vi "code to create file.vi"(0 "queue":refnum<queue>, 2 "Procesar datos en Matlab":bool, 9 "Path":path, 11 "error in (no error)":errorcluster) -> (4 "queue  out":refnum<queue>, 15 "error out":errorcluster)   [LabVIEW 2013]
doc: "This SubVI contain code to create file"
uses:
  bus to create file.ctl
  data simulation bus.ctl
  VoltElectrodo.ctl
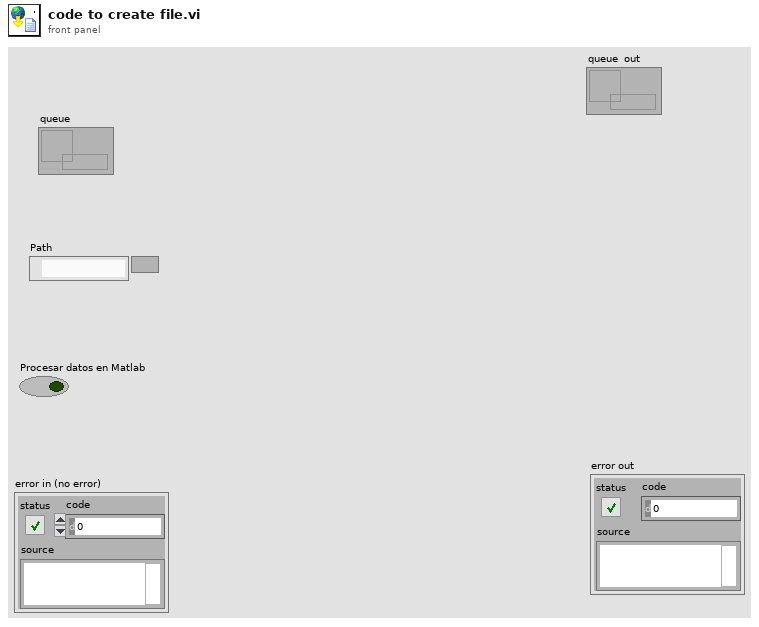
[diagram p1: front panel]
types:
  T1 = typedef "bus to create file.ctl" = cluster{"data simulation":T2, "Time":dbl, "volt":T3}
  T2 = typedef "data simulation bus.ctl" = cluster{"Flujo pulpa ":dbl, "Flujo agua lavado":dbl, "Flujo aire":dbl, "Flujo relave":dbl, "Altura capa de espuma":dbl, "Gas holdup":dbl, "% apertura valvula aire":dbl, "ref pulp":dbl}
  T3 = typedef "VoltElectrodo.ctl" = cluster{"V1":dbl, "V2":dbl, "V3":dbl, "V4":dbl, "V5":dbl, "V6":dbl, "V7":dbl, "V8":dbl}
  T4 = enum16{"open", "replace", "create", "open or create", "replace or create", "replace or create with confirmation"}
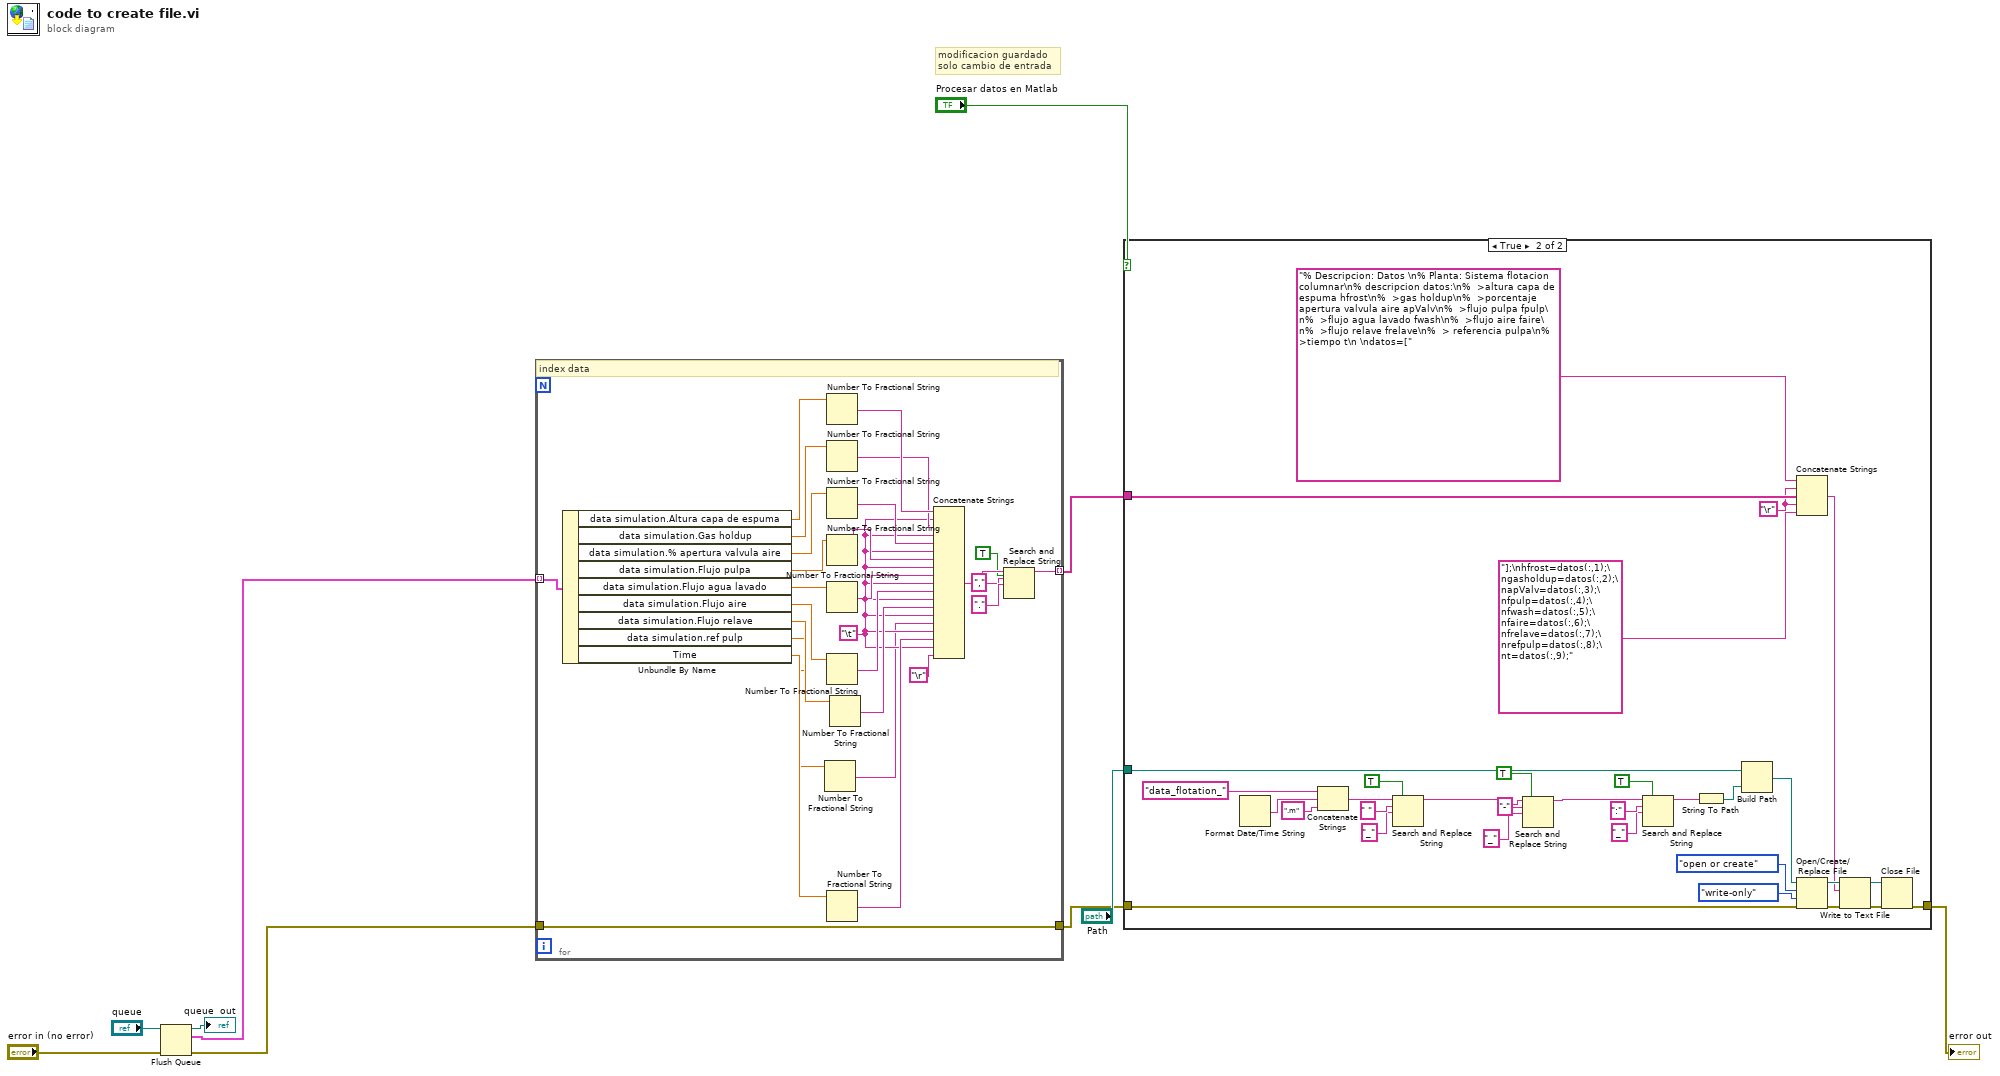
[diagram p0: block diagram]
diagram:
  # "modificacion guardado\nsolo cambio de entrada"
  n1 = Flush Queue(queue="queue", error in (no error)="error in (no error)") -> (queue out=→"queue  out":refnum<queue>, remaining elements=w6:T1[], error out=w3:errorcluster)
  n2 = for {
    tunnel: w6 -> [w30] mode=indexing
    tunnel: [w26] -> w5 mode=indexing
    tunnel: w3 -> [w24]
    tunnel: [w24] -> w4
    w12 = "\t"
    # "index data"
    n3 = Unbundle By Name(w30) -> ("data simulation.Altura capa de espuma"=w19:dbl, "data simulation.Gas holdup"=w17:dbl, "data simulation.% apertura valvula aire"=w20:dbl, "data simulation.Flujo pulpa"=w23:dbl, "data simulation.Flujo agua lavado"=w34:dbl, "data simulation.Flujo aire"=w33:dbl, "data simulation.Flujo relave"=w32:dbl, "data simulation.ref pulp"=w14:dbl, "Time"=w15:dbl)
    n4 = Number To Fractional String(number=w14) -> (F-format string=w11:string)  [unwired: 3 in]
    n5 = Number To Fractional String(number=w19) -> (F-format string=w18:string)  [unwired: 3 in]
    n6 = Number To Fractional String(number=w17) -> (F-format string=w16:string)  [unwired: 3 in]
    n7 = Number To Fractional String(number=w20) -> (F-format string=w21:string)  [unwired: 3 in]
    n8 = Number To Fractional String(number=w23) -> (F-format string=w22:string)  [unwired: 3 in]
    n9 = Number To Fractional String(number=w34) -> (F-format string=w37:string)  [unwired: 3 in]
    n10 = Number To Fractional String(number=w33) -> (F-format string=w36:string)  [unwired: 3 in]
    n11 = Number To Fractional String(number=w15) -> (F-format string=w13:string)  [unwired: 3 in]
    n12 = Number To Fractional String(number=w32) -> (F-format string=w35:string)  [unwired: 3 in]
    n13 = Concatenate Strings(w18, w12, w16, w12, w21, w12, w22, w12, w37, w12, w36, w12, w35, w12, w11, w12, w13, w12, "\r") -> (w27:string)
    n14 = Search and Replace String(replace all?=TRUE ("replace all? (F)"), input string=w27, search string=",", replace string="." ("replace string (\"\")")) -> (result string=w26:string)  [unwired: 4 in, 3 out]
  }
  n15 = case shown="True" "Procesar datos en Matlab" {
    tunnel: w4 -> [w38 w70]
    tunnel: [w38 w69] -> w1
    tunnel: w5 -> [_ w68]
    tunnel: "Path" -> [_ w67]
    frame False {
    }
    frame True {
      w59 = "\r"
      n16 = Format Date/Time String() -> (date/time string=w55:string)  [unwired: 3 in]
      n17 = Concatenate Strings("data_flotation_" ("string"), w55, ".m" ("string")) -> (w52:string)
      n18 = Search and Replace String(replace all?=TRUE ("replace all? (F)"), input string=w52, search string=" ", replace string="_" ("replace string (\"\")")) -> (result string=w43:string)  [unwired: 4 in, 3 out]
      n19 = Search and Replace String(replace all?=TRUE ("replace all? (F)"), input string=w43, search string="-", replace string="_" ("replace string (\"\")")) -> (result string=w42:string)  [unwired: 4 in, 3 out]
      n20 = Search and Replace String(replace all?=TRUE ("replace all? (F)"), input string=w42, search string=":", replace string="_" ("replace string (\"\")")) -> (result string=w45:string)  [unwired: 4 in, 3 out]
      n21 = String To Path(string=w45) -> (path=w44:path)
      n22 = Build Path(base path=w67, name or relative path=w44) -> (appended path=w66:path)
      n23 = Concatenate Strings("% Descripcion: Datos \n% Planta: Sistema flotacion columnar\n% descripcion datos:\n%  >altura capa de espuma hfrost\n%  >gas holdup\n%  >porcentaje apertura valvula aire apValv\n%  >flujo pulpa fpulp\n%  >flujo agua lavado fwash\n%  >flujo aire faire\n%  >flujo relave frelave\n%  > referencia pulpa\n%  >tiempo t\n \ndatos=[", w59, w68, w59, "];\nhfrost=datos(:,1);\ngasholdup=datos(:,2);\napValv=datos(:,3);\nfpulp=datos(:,4);\nfwash=datos(:,5);\nfaire=datos(:,6);\nfrelave=datos(:,7);\nrefpulp=datos(:,8);\nt=datos(:,9);" ("string")) -> (w58:string)
      n24 = Open/Create/Replace File(file path (use dialog)=w66, error in=w70, operation (0:open)=T4."open or create", access (0:read/write)=enum16{"read/write", "read-only", "write-only"}."write-only") -> (refnum out=w63:refnum<file>, error out=w62:errorcluster)  [unwired: 2 in, 1 out]
      n25 = Write to Text File(file (use dialog)=w63, text=w58, error in=w62) -> (refnum out=w61:refnum<file>, error out=w60:errorcluster)  [unwired: 1 in, 1 out]
      n26 = Close File(refnum=w61, error in=w60) -> (error out=w69:errorcluster)  [unwired: 1 out]
    }
  }
  "error out" <- w1
